vi "Edit Connector Pane for Wrapper.vi"(0 "vi reference in":refnum<vi>, 11 "error in":errorcluster) -> (4 "vi reference out":refnum<vi>, 15 "error out":errorcluster)   [LabVIEW 2021, in "Converter.lvlib"]
uses:
  Converter.lvlib
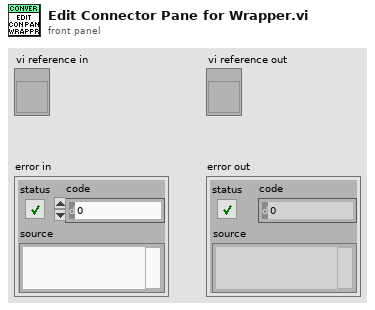
[diagram p1: front panel]
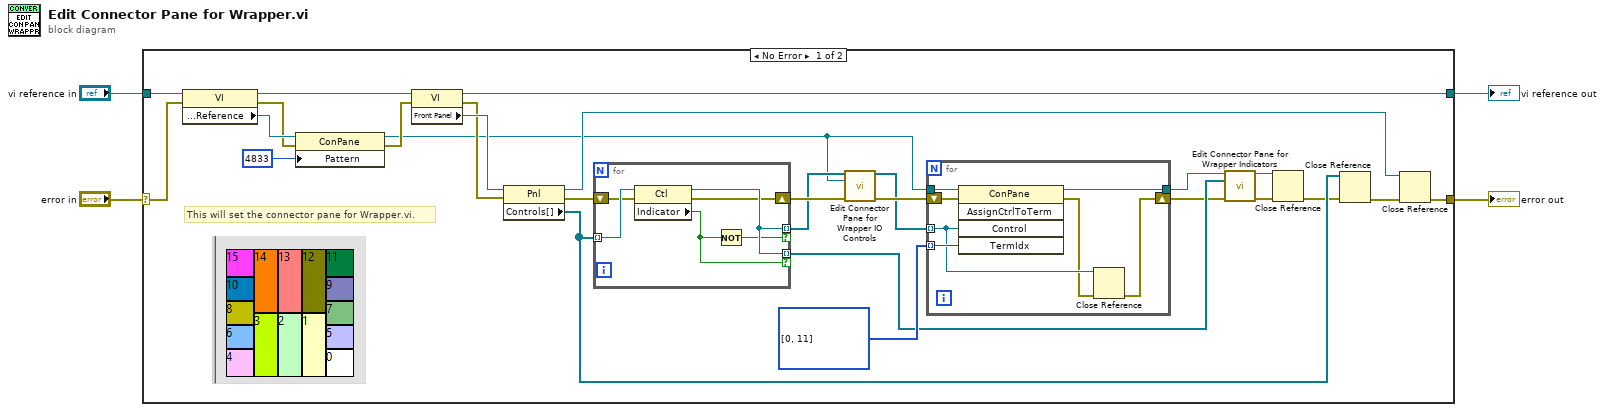
[diagram p0: block diagram]
diagram:
  n1 = case shown="No Error" "error in" {
    selector: "error in" -> [w20 w46]
    tunnel: [w15 w46] -> w4
    tunnel: "vi reference in" -> [w14 w45]
    tunnel: [w13 w45] -> w1
    frame No Error {
      # "This will set the connector pane for Wrapper.vi."
      n2 = property class="VI"(reference=w14, error in=w20) -> (reference out=w31:refnum<vi>, error out=w26:errorcluster, "Connector Pane:Reference"=w28:refnum<vi>)
      n3 = property class="ConPane"(reference=w28, error in=w26, "Pattern"=u32 4833) -> (reference out=w5:refnum<vi>, error out=w27:errorcluster)
      n4 = property class="VI"(reference=w31, error in=w27) -> (reference out=w13:refnum<vi>, error out=w29:errorcluster, "Front Panel"=w30:refnum<vi>)
      n5 = property class="Pnl"(reference=w30, error in=w29) -> (reference out=w19:refnum<vi>, error out=w12:errorcluster, "Controls[]"=w18:refnum<vi>[])
      n6 = for {
        tunnel: w18 -> [w44] mode=indexing
        shift-right: [w40] -> w11
        shift-left: w12 -> [w43]
        tunnel: [w42] -> w23 mode=indexing if=w39
        tunnel: [w42] -> w9 mode=indexing if=w41
        n7 = property class="Ctl"(reference=w44, error in=w43) -> (reference out=w42:refnum<vi>, error out=w40:errorcluster, "Indicator"=w39:bool)
        n8 = Not(x=w39) -> (.not. x?=w41:bool)
      }
      n9 = call "Edit Connector Pane for Wrapper IO Controls.vi"("controls in[]"=w9, "con pane in"=w5, "error in"=w11) -> ("other controls[]"=w8:refnum<vi>[], "error out"=w10:errorcluster)  [unwired: 11 in]
      n10 = for {
        tunnel: w8 -> [w35] mode=indexing
        tunnel: u32[] [0, 11] ("Terminal Index") -> [w38] mode=indexing
        tunnel: w5 -> [w37]
        shift-right: [w34] -> w22
        shift-left: w10 -> [w36]
        tunnel: [w33] -> w24
        n11 = invoke class="ConPane" method="AssignCtrlToTerm"(reference=w37, error in=w36, "Control"=w35, "TermIdx"=w38) -> (reference out=w33:refnum<vi>, error out=w32:errorcluster)  [unwired: 1 in, 3 out]
        n12 = Close Reference(reference=w35, error in (no error)=w32) -> (error out=w34:errorcluster)
      }
      n13 = call "Edit Connector Pane for Wrapper Indicators.vi"("con pane in"=w24, "indicators in[]"=w23, "error in"=w22) -> ("con pane out"=w7:refnum<vi>, "error out"=w21:errorcluster)  [unwired: 11 in]
      n14 = Close Reference(reference=w7, error in (no error)=w21) -> (error out=w17:errorcluster)
      n15 = Close Reference(reference=w18, error in (no error)=w17) -> (error out=w16:errorcluster)
      n16 = Close Reference(reference=w19, error in (no error)=w16) -> (error out=w15:errorcluster)
    }
    frame Error {
    }
  }
  "error out" <- w4
  "vi reference out" <- w1
